vi "Open HTML Report in Browser.vi"(8 "error in (no error)":errorcluster, 11 "report in":T1) -> (0 "error out":errorcluster, 2 "temporary HTML file created":path, 3 "report out":T1)   [LabVIEW 2020]
doc: "Displays an HTML report in the default Web browser. The data type you wire to the <B>report in</B> input determines the polymorphic instance to use. You cannot use this VI with standard reports."
uses:
  <vilib>/Utility/NIReport.llb/Generate Report Object Reference.ctl
  <vilib>/Utility/NIReport.llb/NI_report.lvclass
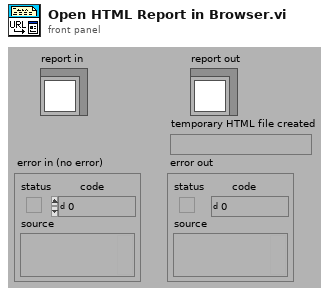
[diagram p1: front panel]
types:
  T1 = typedef "Generate Report Object Reference.ctl" = refnum<class "NI_report.lvclass">
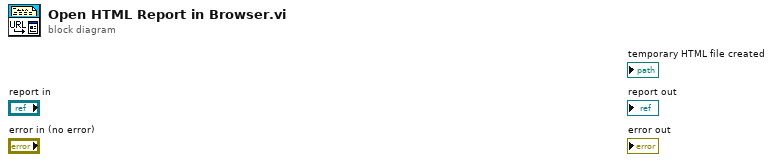
[diagram p0: block diagram]
diagram:
